vi "runscenario parse Query.vi"(11 "Query as Key/Value (empty)":T1) -> (2 "ANDed Condition Logic":string, 3 "Search Parameters":T2[](array[typedef]))   [LabVIEW 2011]
uses:
  server/DataFinder/Datafinder Query.ctl
  server/DataFinder/eSearch Types.ctl
  server/DataFinder/DataFinder Comparisons.ctl
  Addons/internet/utils/keyedarr.llb/Keyed Array.ctl
  Addons/internet/utils/strutil.llb/Case Matching.ctl
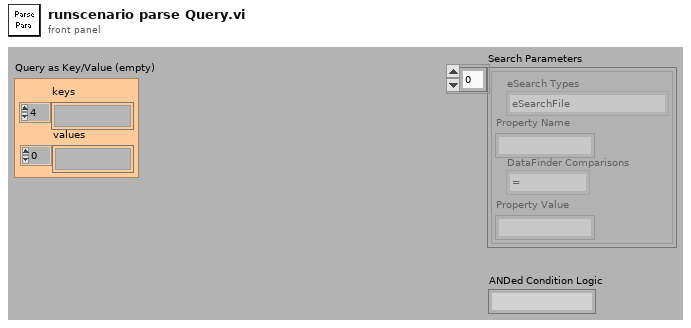
[diagram p1: front panel]
types:
  T1 = typedef "Keyed Array.ctl" = cluster{"keys":string[], "values":string[]}
  T2 = typedef "Datafinder Query.ctl" = cluster{"eSearch Types":T3, "Property Name":string, "DataFinder Comparisons":T4, "Property Value":string}
  T3 = typedef "eSearch Types.ctl" = enum16{"eSearchFile", "eSearchChannelGroup", "eSearchChannel"}
  T4 = typedef "DataFinder Comparisons.ctl" = enum16{"=", "<>", "<", "<=", ">", ">="}
  T5 = typedef "Case Matching.ctl" = enum16{"a != A", "a == A", "system"}
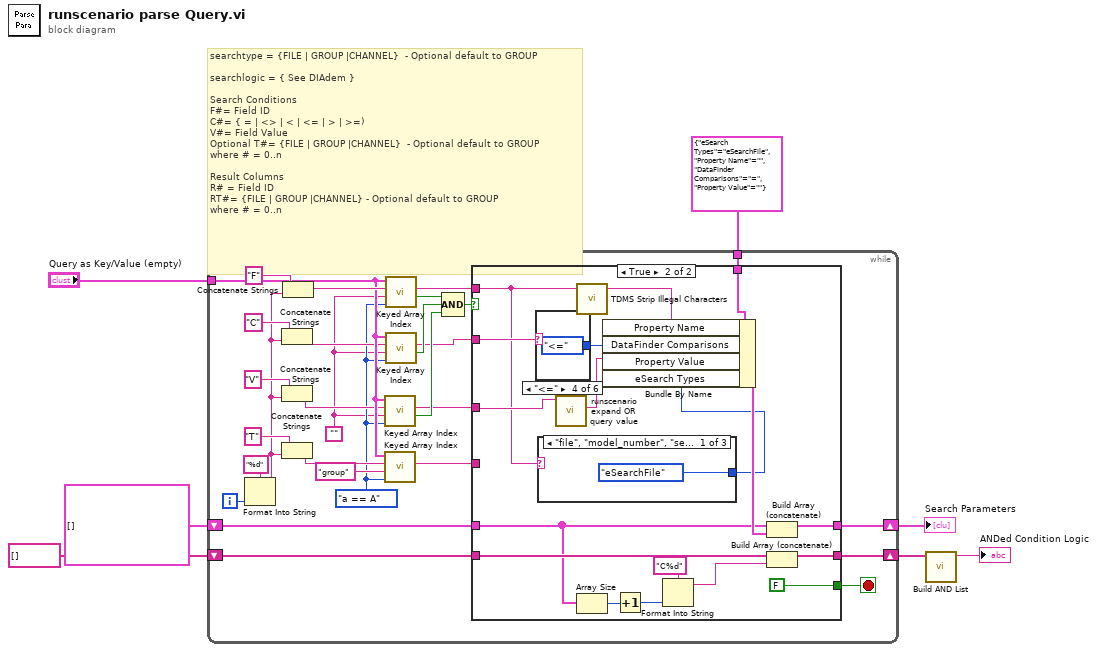
[diagram p0: block diagram]
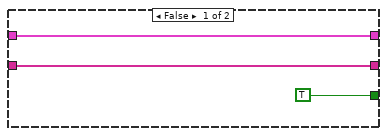
[diagram p2: hidden frame]
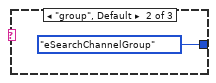
[diagram p3: hidden frame]
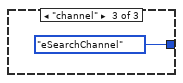
[diagram p4: hidden frame]
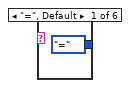
[diagram p5: hidden frame]
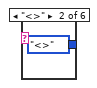
[diagram p6: hidden frame]
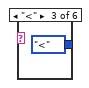
[diagram p7: hidden frame]
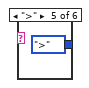
[diagram p8: hidden frame]
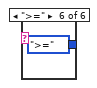
[diagram p9: hidden frame]
diagram:
  # "searchtype = {FILE | GROUP |CHANNEL}  - Optional default to GROUP \n\nsearchlogic = { See DIAdem }\n\nSearch Conditions\nF#= Field ID\nC#= { = | <> | < | <= | > | >=)\nV#= Field Value\nOptional T#= {FILE | GROUP |CHANNEL}  - Optional default to GROUP \nwhere # = 0..n\n\nResult Columns\nR# = Field ID\nRT#= {FILE | GROUP |CHANNEL} - Optional default to GROUP \nwhere # = 0..n"
  n1 = while {
    tunnel: "Query as Key/Value (empty)" -> [w29]
    shift-right: [w16] -> w4
    shift-left: T2[] [] ("initialized array") -> [w18]
    tunnel: T2 {"eSearch Types"=enum."eSearchFile", "Property Name"="", "DataFinder Comparisons"=enum."=", "Property Value"=""} ("Data Finder Parameters") -> [w11]
    shift-right: [w9] -> w6
    shift-left: string[] [] ("initialized array") -> [w8]
    i -> [w10]
    stop <- w25 stop-if-true
    w13 = ""
    w23 = Case_Matching."a == A" ("case matching (sensitive)")
    n2 = Format Into String(format string="%d", w10) -> (resulting string=w24:string)  [unwired: 2 in, 1 out]
    n3 = Concatenate Strings("C" ("key"), w24) -> (w28:string)
    n4 = Concatenate Strings("V" ("key"), w24) -> (w27:string)
    n5 = Concatenate Strings("T" ("key"), w24) -> (w26:string)
    n6 = Concatenate Strings("F" ("key"), w24) -> (w30:string)
    n7 = call "Keyed Array Index.vi"("case matching (sensitive)"=w23, "default value"=w13, "key"=w27, "array in"=w29) -> ("valid key"=w20:bool, "value"=w14:string)  [unwired: 2 out]
    n8 = call "Keyed Array Index.vi"("case matching (sensitive)"=w23, "default value"="group" ("key"), "key"=w26, "array in"=w29) -> ("value"=w12:string)  [unwired: 3 out]
    n9 = call "Keyed Array Index.vi"("case matching (sensitive)"=w23, "default value"=w13, "key"=w30, "array in"=w29) -> ("valid key"=w22:bool, "value"=w17:string)  [unwired: 2 out]
    n10 = call "Keyed Array Index.vi"("case matching (sensitive)"=w23, "default value"=w13, "key"=w28, "array in"=w29) -> ("valid key"=w21:bool, "value"=w15:string)  [unwired: 2 out]
    n11 = Compound Arithmetic op=AND(w22, w21, w20) -> (w19:bool)
    n12 = case shown="True" w19 {
      tunnel: [TRUE FALSE] -> w25
      tunnel: w18 -> [w38 w45]
      tunnel: [w38 w56] -> w16
      tunnel: w11 -> [_ w55]
      tunnel: w17 -> [_ w40]
      tunnel: w15 -> [_ w52]
      tunnel: w14 -> [_ w49]
      tunnel: w12 -> [_ _]
      tunnel: [w37 w47] -> w9
      tunnel: w8 -> [w37 w46]
      frame False {
      }
      frame True {
        n13 = case shown="\"<=\"" w52 {
          tunnel: [DataFinder_Comparisons."=" ("DataFinder Comparisons") DataFinder_Comparisons."<>" ("DataFinder Comparisons") DataFinder_Comparisons."<" ("DataFinder Comparisons") DataFinder_Comparisons."<=" ("DataFinder Comparisons") DataFinder_Comparisons.">" ("DataFinder Comparisons") DataFinder_Comparisons.">=" ("DataFinder Comparisons")] -> w53
          frame "=", Default {
          }
          frame "<>" {
          }
          frame "<" {
          }
          frame "<=" {
          }
          frame ">" {
          }
          frame ">=" {
          }
        }
        n14 = case shown="\"file\", \"model_number\", \"serial_number\", \"TEST_TYPE\"" w40 {
          tunnel: [eSearch_Types."eSearchFile" ("eSearch Type") eSearch_Types."eSearchChannelGroup" ("eSearch Type") eSearch_Types."eSearchChannel" ("eSearch Type")] -> w51
          frame "file", "model_number", "serial_number", "TEST_TYPE" {
          }
          frame "group", Default {
          }
          frame "channel" {
          }
        }
        n15 = call "runscenario expand OR query value.vi"("Value String"=w49) -> ("Value OR String"=w48:string)  [unwired: 10 out]
        n16 = call "TDMS Strip Illegal Characters.vi"("String"=w40) -> ("Legal String"=w50:string)  [unwired: 4 out]
        n17 = Array Size(array=w45) -> (size(s)=w44:i32)
        n18 = Bundle By Name(cluster=w55, "Property Name"=w50, "DataFinder Comparisons"=w53, "Property Value"=w48, "eSearch Types"=w51) -> (w54:T2)
        n19 = Increment(x=w44) -> (x+1=w43:i32)
        n20 = Format Into String(format string="C%d", w43) -> (resulting string=w42:string)  [unwired: 2 in, 1 out]
        n21 = Build Array (concatenate)(w45, w54) -> (w56:T2[])
        n22 = Build Array (concatenate)(w46, w42) -> (w47:string[])
      }
    }
  }
  "Search Parameters" <- w4
  n23 = call "Build AND List.vi"("String Array"=w6) -> ("AND String"=→"ANDed Condition Logic":string)  [unwired: 10 out]
